vi "cpx from fifo to array.vi"(6 "channel 1":u64[](array[numeric]), 9 "channel 2":u64[](array[numeric]), 10 "channel 3":u64[](array[numeric]), 11 "channel 4":u64[](array[numeric])) -> (3 "Array":cdb[](array[numeric]))   [LabVIEW 2020]
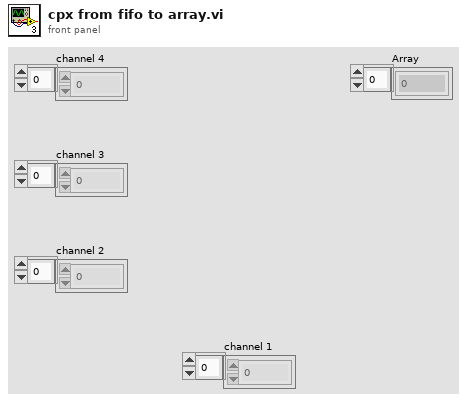
[diagram p1: front panel]
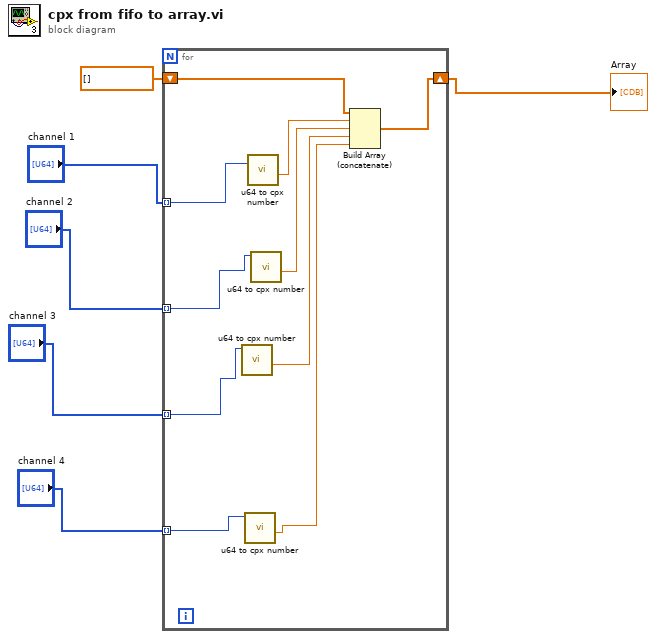
[diagram p0: block diagram]
diagram:
  n1 = for {
    tunnel: "channel 4" -> [w12] mode=indexing
    shift-right: [w14] -> w6
    shift-left: cdb[] [] -> [w15]
    tunnel: "channel 1" -> [w16] mode=indexing
    tunnel: "channel 2" -> [w10] mode=indexing
    tunnel: "channel 3" -> [w11] mode=indexing
    n2 = call "u64 to cpx number.vi"("Numeric"=w11) -> ("x + iy"=w8:cdb)  [unwired: 10 in]
    n3 = call "u64 to cpx number.vi"("Numeric"=w12) -> ("x + iy"=w7:cdb)  [unwired: 10 in]
    n4 = call "u64 to cpx number.vi"("Numeric"=w16) -> ("x + iy"=w13:cdb)  [unwired: 10 in]
    n5 = call "u64 to cpx number.vi"("Numeric"=w10) -> ("x + iy"=w9:cdb)  [unwired: 10 in]
    n6 = Build Array (concatenate)(w15, w13, w9, w8, w7) -> (w14:cdb[])
  }
  "Array" <- w6
